vi "tb_00-i.vi"(0 "Etude":T1, 1 "Aff ?":bool, 5 "VS":T3, 7 "ent-2D":string[][](array[string]), 9 "do-2D":string[][](array[string]), 11 "tb in ?":bool[](array[boolean])) -> (4 "Etude":T1, 6 "VS":T3, 8 "ent-2D 2":string[][](array[string]), 10 "do-2D":string[][](array[string]), 12 "X":string[](array[string]), 13 "xc-ent":string, 14 "xc-lib":string, 15 "tb in ?":bool[](array[boolean]))   [LabVIEW 2010, in "lv_04.lvlib"]
uses:
  lv_04/commandes/cX.ctl
  lv_04/commandes/cSTA_varid.ctl
  lv_04/commandes/c_TDMS_ch_variable.ctl
  lv_04/commandes/c_TDMS_ch_donnees.ctl
  lv_04/commandes/c0-var-n.ctl
  lv_04/commandes/cSTA_num_do_cr.ctl
  lv_04/commandes/c02-do-num.ctl
  lv_04/commandes/c04-stat-num.ctl
  lv_04/commandes/cSTA_txt_do_cr.ctl
  lv_04/commandes/c02-do-txt.ctl
  lv_04/commandes/c04-stat-txt.ctl
  lv_04/commandes/cSTA_dist.ctl
  lv_04/commandes/c03-dist-S.ctl
  lv_04/commandes/c0-dist-xy.ctl
  lv_04/commandes/c03-dist-T.ctl
  lv_04/commandes/c03-dist-SPC.ctl
  lv_04/commandes/c_etude.ctl
  lv_02/p_5E_ch_loi.ctl
  lv_01/type format.ctl
  lv_04/lv_04.lvlib
  lv_01/lv_01.lvlib
  lv_02/lv_02.lvlib
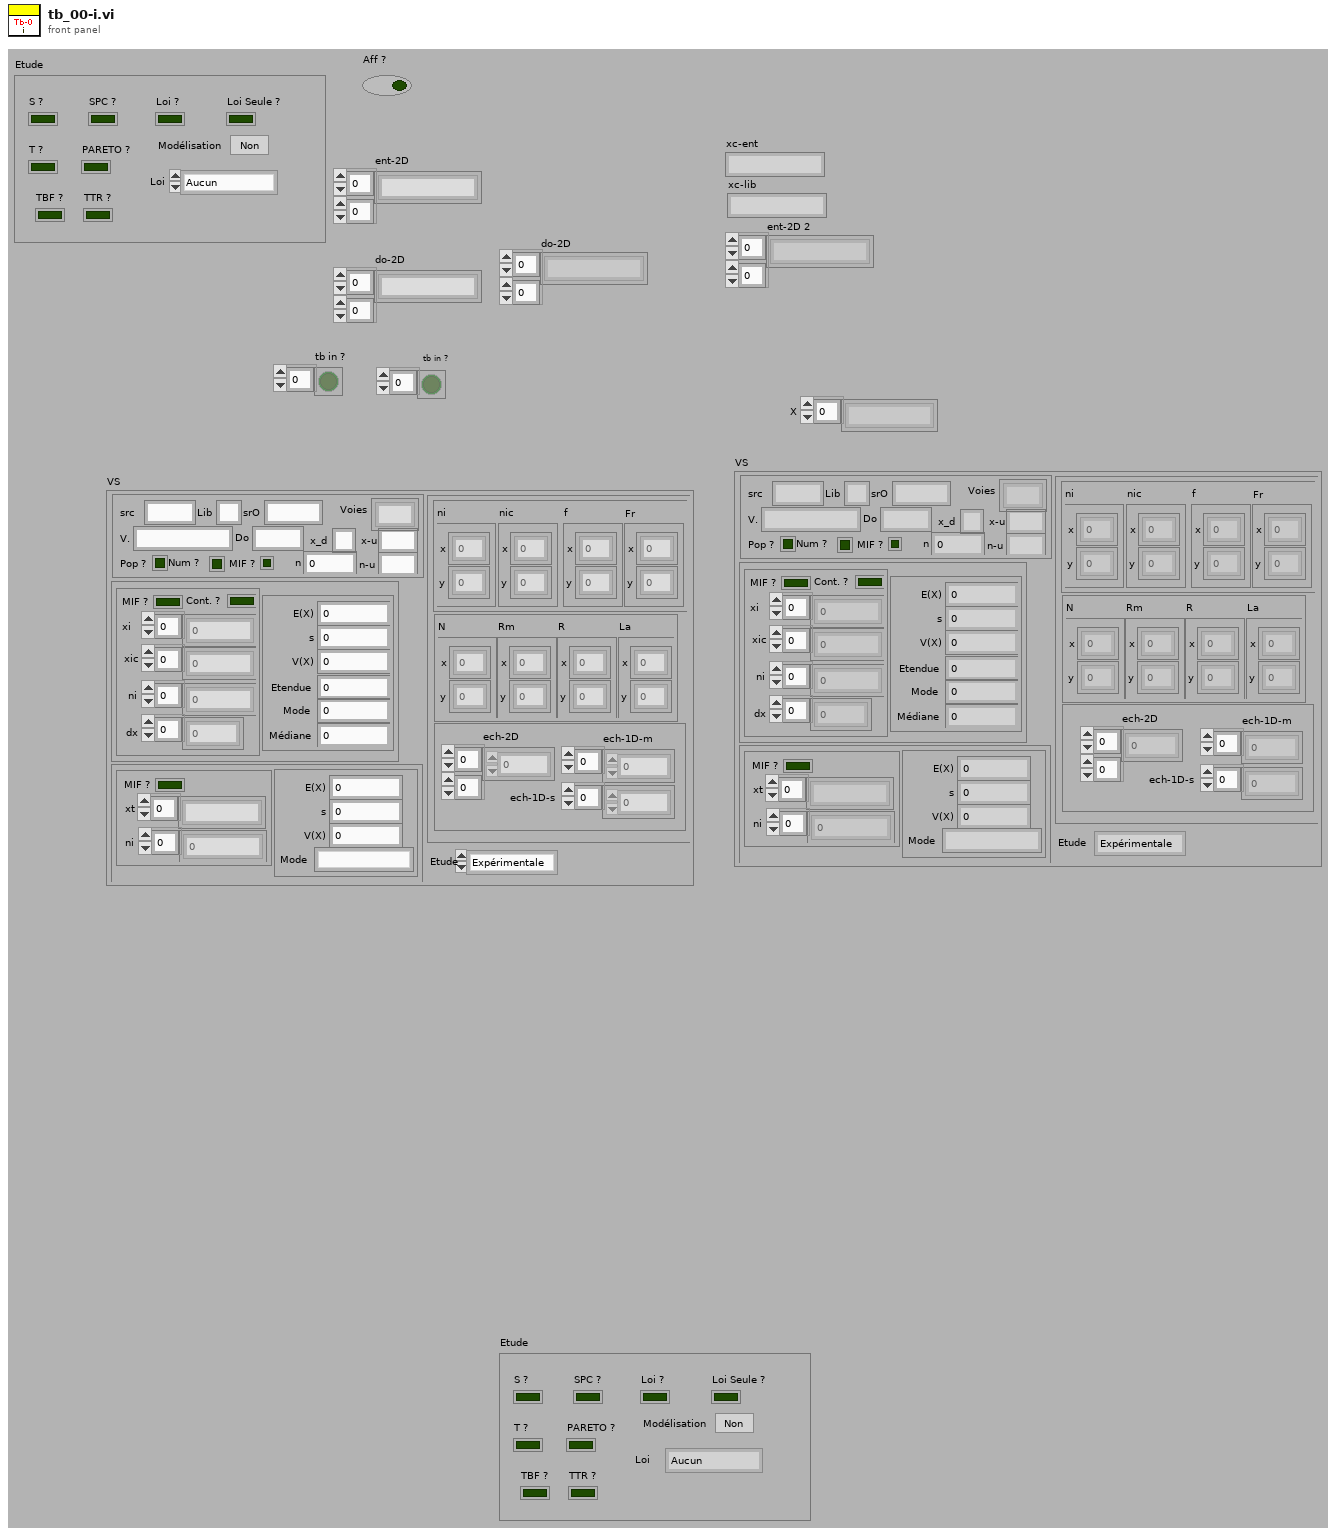
[diagram p1: front panel]
types:
  T1 = typedef "lv_04.lvlib/c_etude.ctl" = cluster{"T ?":bool, "S ?":bool, "SPC ?":bool, "PARETO ?":bool, "TBF ?":bool, "TTR ?":bool, "Loi ?":bool, "Loi Seule ?":bool, "Modélisation":bool, "Loi":T2}
  T2 = typedef "lv_02.lvlib/p_5E_ch_loi.ctl" = enum16{"Aucun", "Normale", "Aucun2", "Aucun3", "Binômial", "Poisson", "Exponentiel", "Weibull", "Rang médian"}
  T3 = typedef "lv_04.lvlib/cX.ctl" = cluster{"src":T4, "num":T8, "txt":T11, "dist":T14, "Etude":enum16{"Expérimentale", "Modèle"}}
  T4 = typedef "lv_04.lvlib/cSTA_varid.ctl" = cluster{"src":string, "Lib":string, "srO":string, "V.":T5, "Voies":string[], "Do":T6, "n":T7, "Num ?":bool, "Pop ?":bool, "x_d":string, "x-u":string, "n-u":string, "MIF ?":bool}
  T5 = typedef "lv_04.lvlib/c_TDMS_ch_variable.ctl" = string
  T6 = typedef "lv_04.lvlib/c_TDMS_ch_donnees.ctl" = string
  T7 = typedef "lv_04.lvlib/c0-var-n.ctl" = i32
  T8 = typedef "lv_04.lvlib/cSTA_num_do_cr.ctl" = cluster{"do":T9, "sta":T10}
  T9 = typedef "lv_04.lvlib/c02-do-num.ctl" = cluster{"MIF ?":bool, "Cont. ?":bool, "xi":dbl[], "xic":dbl[], "ni":u32[], "dx":dbl[]}
  T10 = typedef "lv_04.lvlib/c04-stat-num.ctl" = cluster{"E(X)":dbl, "s":dbl, "V(X) ":dbl, "Etendue":dbl, "Mode":dbl, "Médiane":dbl}
  T11 = typedef "lv_04.lvlib/cSTA_txt_do_cr.ctl" = cluster{"do":T12, "sta":T13}
  T12 = typedef "lv_04.lvlib/c02-do-txt.ctl" = cluster{"xt":string[], "ni":dbl[], "MIF ?":bool}
  T13 = typedef "lv_04.lvlib/c04-stat-txt.ctl" = cluster{"E(X)":dbl, "s":dbl, "V(X) ":dbl, "Mode":string}
  T14 = typedef "lv_04.lvlib/cSTA_dist.ctl" = cluster{"S":T15, "T":T17, "spc":T18}
  T15 = typedef "lv_04.lvlib/c03-dist-S.ctl" = cluster{"nic":T16, "f":T16, "Fr":T16, "ni":T16}
  T16 = typedef "lv_04.lvlib/c0-dist-xy.ctl" = cluster{"x":dbl[], "y":dbl[]}
  T17 = typedef "lv_04.lvlib/c03-dist-T.ctl" = cluster{"N":T16, "Rm":T16, "R":T16, "La":T16}
  T18 = typedef "lv_04.lvlib/c03-dist-SPC.ctl" = cluster{"ech-2D":dbl[][], "ech-1D-m":dbl[], "ech-1D-s":dbl[]}
  T19 = typedef "lv_01.lvlib/type format.ctl" = enum16{"X (dbl)", "P (Proba)", "N (entier)", "S (Scient.)"}
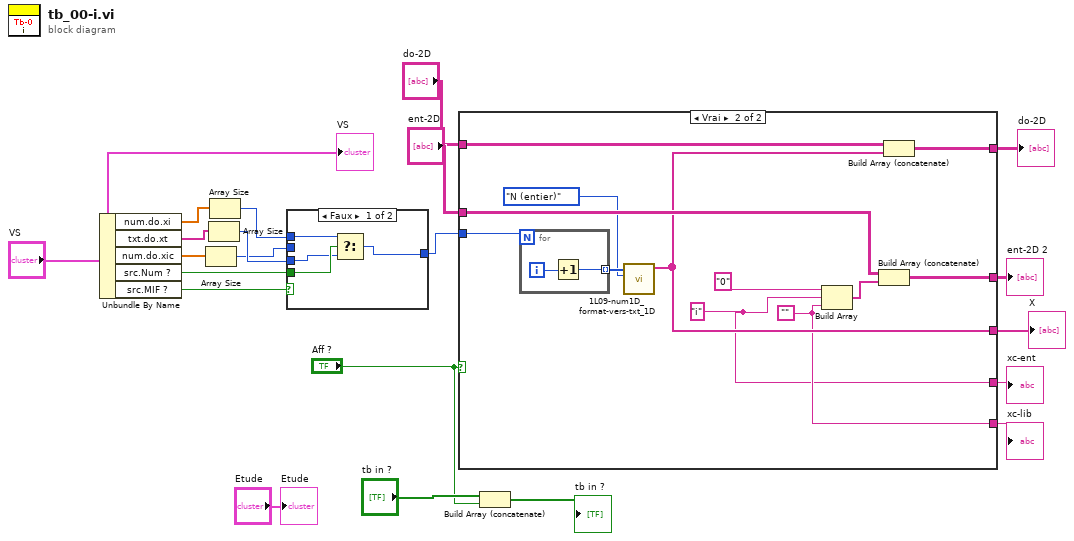
[diagram p0: block diagram]
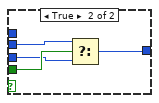
[diagram p2: hidden frame]
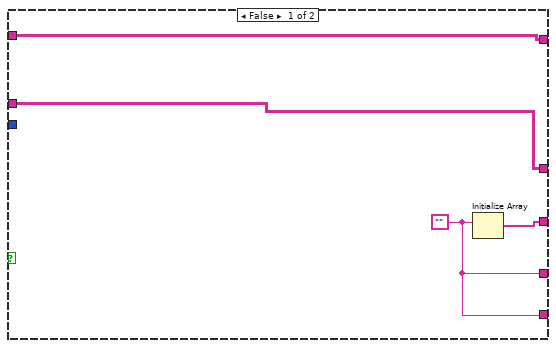
[diagram p3: hidden frame]
diagram:
  n1 = Unbundle By Name("VS") -> ("num.do.xi"=w10:dbl[], "txt.do.xt"=w11:string[], "num.do.xic"=w12:dbl[], "src.Num ?"=w5:bool, "src.MIF ?"=w4:bool)
  n2 = Array Size(array=w12) -> (size(s)=w7:i32)
  n3 = Array Size(array=w11) -> (size(s)=w8:i32)
  n4 = Array Size(array=w10) -> (size(s)=w9:i32)
  n5 = case shown="Faux" w4 {
    tunnel: w9 -> [w23 _]
    tunnel: w8 -> [w22 w27]
    tunnel: w7 -> [_ w28]
    tunnel: w5 -> [w24 w29]
    tunnel: [w25 w26] -> w6
    frame False {
      n6 = Select(t=w23, s=w24, f=w22) -> (s? t:f=w25:i32)
    }
    frame True {
      n7 = Select(t=w28, s=w29, f=w27) -> (s? t:f=w26:i32)
    }
  }
  n8 = case shown="Vrai" "Aff ?" {
    tunnel: [w30 w34] -> w3
    tunnel: [w30 w36] -> w2
    tunnel: "ent-2D" -> [w32 w44]
    tunnel: [w32 w42] -> w1
    tunnel: "do-2D" -> [w33 w41]
    tunnel: [w31 w37] -> w17
    tunnel: [w33 w40] -> w16
    tunnel: w6 -> [_ w35]
    frame False {
      w30 = ""
      n9 = Initialize Array(w30) -> (w31:string[])  [unwired: 1 in]
    }
    frame True {
      w34 = "i" ("élément")
      w36 = ""
      n10 = for {
        N: w35 -> [_]
        tunnel: [w46] -> w39 mode=indexing
        i -> [w47]
        n11 = Increment(x=w47) -> (x+1=w46:i32)
      }
      n12 = call "1L09-num1D_format-vers-txt_1D.vi"("type"=type_format."N (entier)", "1D( num)"=w39) -> ("1D (ch)"=w37:string[])  [unwired: 7 in]
      n13 = Build Array("0", w34, w36) -> (w43:string[])
      n14 = Build Array (concatenate)(w44, w43) -> (w42:string[][])
      n15 = Build Array (concatenate)(w41, w37) -> (w40:string[][])
    }
  }
  "X" <- w17
  "do-2D" <- w16
  "xc-ent" <- w3
  "xc-lib" <- w2
  "ent-2D 2" <- w1
  n16 = Build Array (concatenate)("tb in ?", "Aff ?") -> (→"tb in ?":bool[])
  "VS" <- "VS"
  "Etude" <- "Etude"
